vi "generate_galvo_voltages_from_fifo.vi"(0 "resonant trigger":bool, 1 "counter cluster in":T5, 2 "stim duration":u16=20, 3 "tracking settings":T1, 4 "scan specification":T4, 5 "scanning":bool, 6 "tracking":bool, 7 "x-y phase shift (*2^16/2*pi)":u16=16384, 9 "stim delay":i16=5) -> (10 "stim light window":bool, 11 "trigger diagnostics":T2, 12 "update tracking?":T3, 13 "counting photons?":bool, 14 "DAC voltages":T6 {"pockels" max=4095 step=1; "y" max=4095 step=1; "x" max=4095 step=1}, 15 "counter cluster out":T5, 17 "new circle":bool, 18 "fly-back acquisition phase?":bool, 19 "acquire?":bool)   [LabVIEW 2010]
uses:
  common_typedefs/DAC_voltage_tagResonantr.ctl
  counter_cluster_tagResonant.ctl
  scan_specification_tagResonant.ctl
  FPGA tracking/polar tracking settings.ctl
  <vilib>/rvi/DataTransferAndStorage/Container/XNode/niFpgaContainer.xnode
  <vilib>/rvi/DataTransferAndStorage/Container/Common/niFpgaContainerMethod.ctl
  <vilib>/rvi/DataTransferAndStorage/Container/Common/niFpgaTransferTypeControl.ctl
  <vilib>/rvi/Analysis/common/FxpNativeNode/niFpgaFxpNative.xnode
  <vilib>/rvi/interface/RandomDataEmulation/nirviRandomDataFPGAFIFO.vi
  <vilib>/rvi/interface/RandomDataEmulation/niFpgaRandomDataHandleErrors.vi
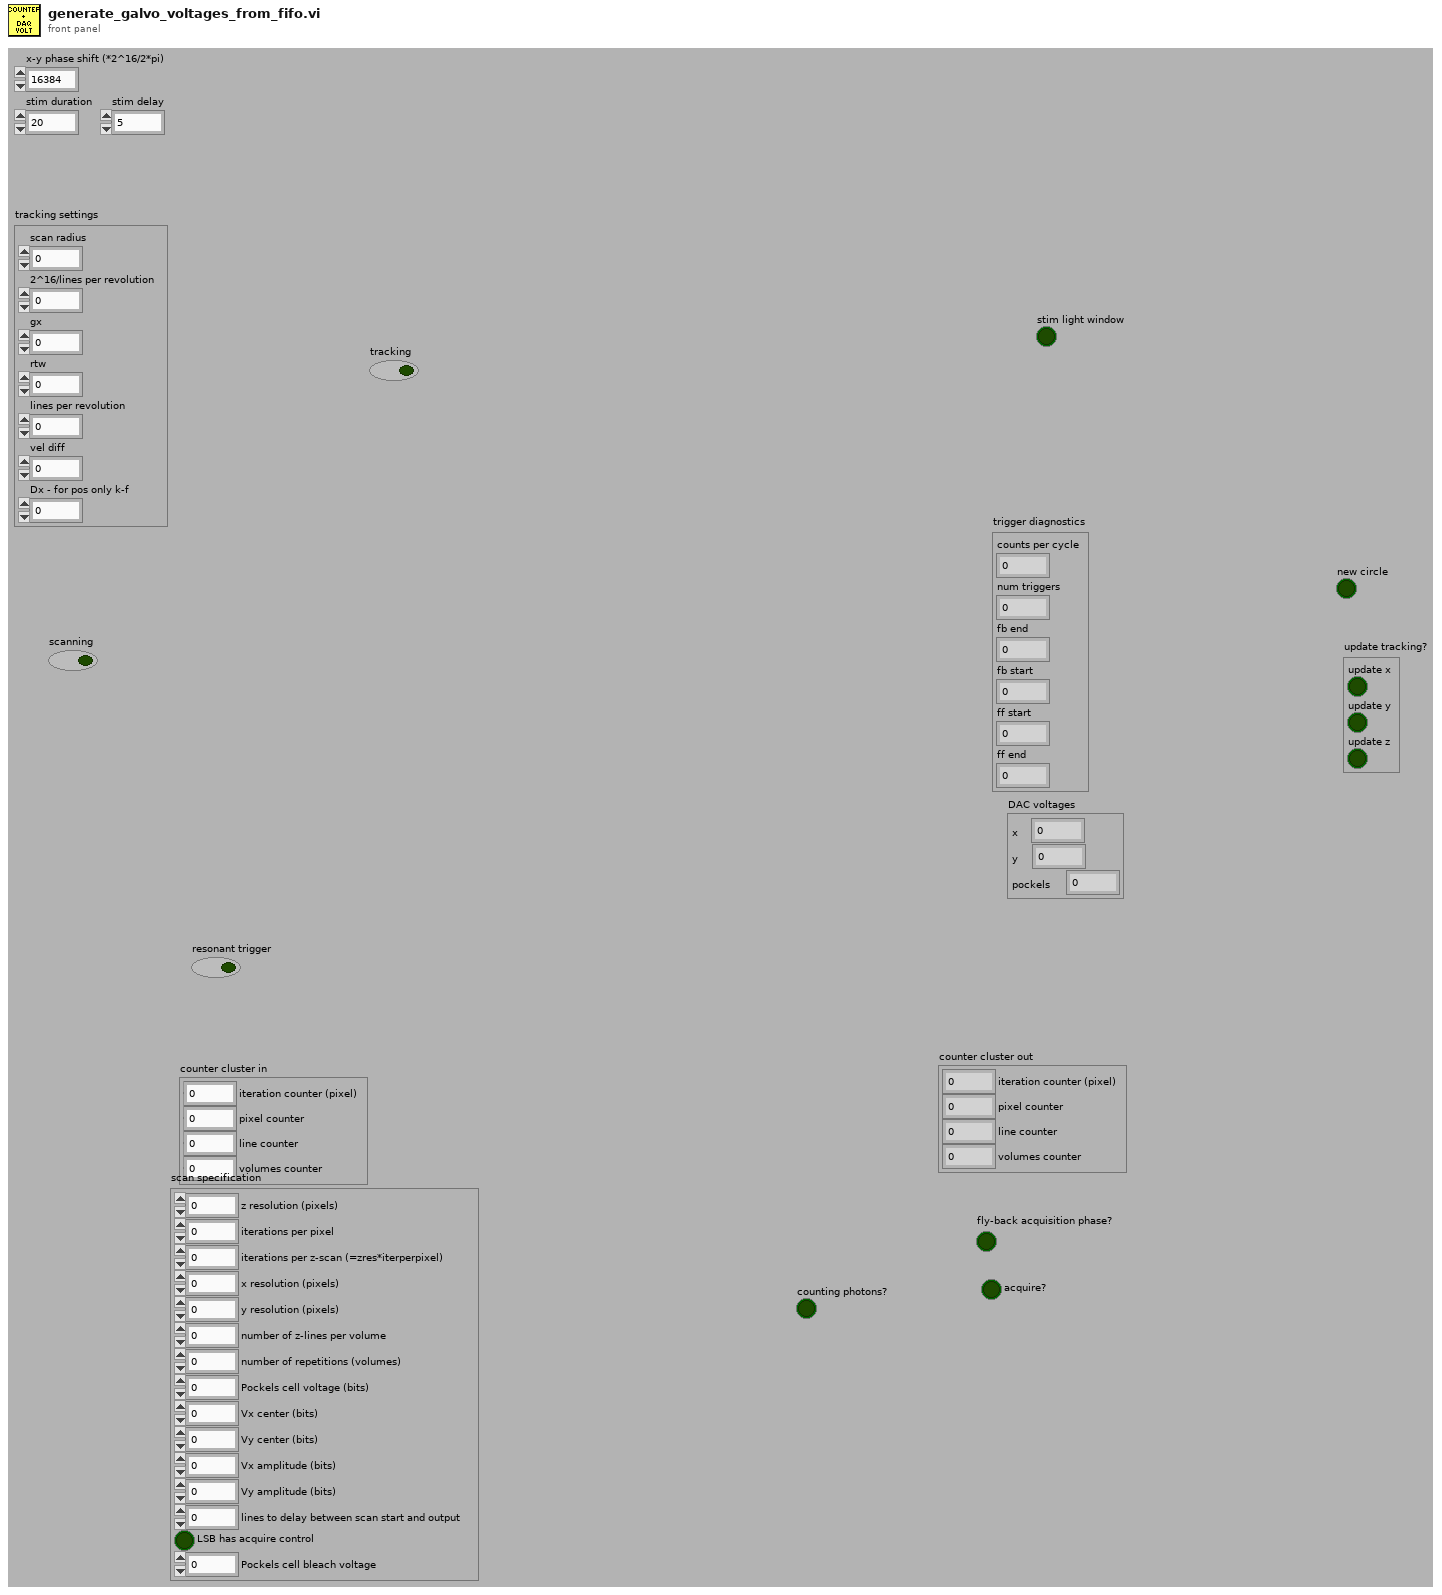
[diagram p1: front panel]
types:
  T1 = typedef "polar tracking settings.ctl" = cluster{"scan radius":u16, "2^16/lines per revolution":u16, "gx":fxp<+,16,8>, "rtw":fxp<+,16,26>, "lines per revolution":u8, "vel diff":fxp<+,24,-22>, "Dx - for pos only k-f":fxp<+,32,19>}
  T2 = cluster{"counts per cycle":u16, "num triggers":u32, "fb end":u16, "fb start":u16, "ff start":u16, "ff end":u16}
  T3 = cluster{"update x":bool, "update y":bool, "update z":bool}
  T4 = typedef "scan_specification_tagResonant.ctl" = cluster{"z resolution (pixels)":u16, "iterations per pixel":u16, "iterations per z-scan (=zres*iterperpixel)":u16, "x resolution (pixels)":u16, "y resolution (pixels)":u16, "number of z-lines per volume":u16, "number of repetitions (volumes)":i32, "Pockels cell voltage (bits)":i16, "Vx center (bits)":i16, "Vy center (bits)":i16, "Vx amplitude (bits)":i16, "Vy amplitude (bits)":i16, "lines to delay between scan start and output":u16, "LSB has acquire control":bool, "Pockels cell bleach voltage":i16}
  T5 = typedef "counter_cluster_tagResonant.ctl" = cluster{"iteration counter (pixel)":u16, "pixel counter":u16, "line counter":i16, "volumes counter":u16}
  T6 = typedef "DAC_voltage_tagResonantr.ctl" = cluster{"x":i16, "y":i16, "pockels":i16}
  T7 = typedef "niFpgaContainerMethod.ctl" = enum16{"<none>", "write", "read", "clear", "getNumberOfElementsToWrite", "getNumberOfElementsToRead", "enable", "disable", "flushAndDisable", "getStreamState", "readA", "readB", "dramWrite", "dramWriteWithByteEnables", "dramRequestData", "dramRetrieveData"}
  T8 = typedef "niFpgaTransferTypeControl.ctl" = enum16{"Target-Scoped", "Host to Target - DMA", "Target to Host - DMA", "Peer to Peer Reader", "Peer to Peer Writer", "Bidirectional"}
  T9 = cluster{"crossing":bool, "crossing":bool, "crossing":bool}
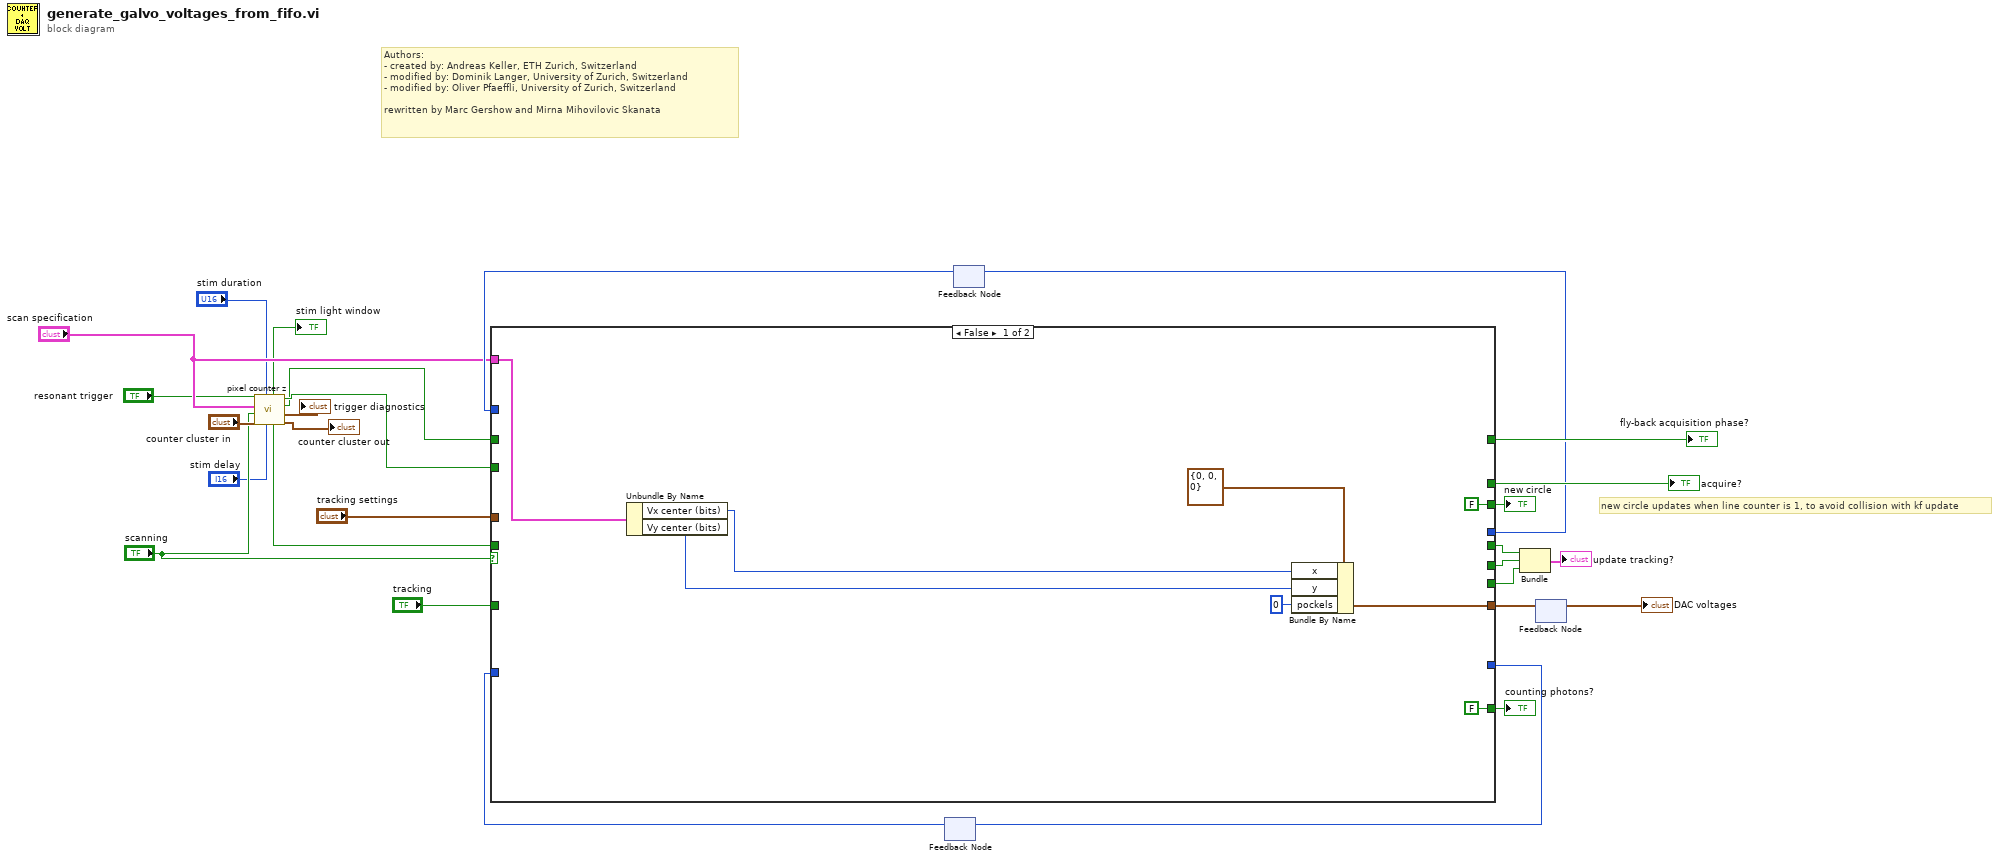
[diagram p0: block diagram]
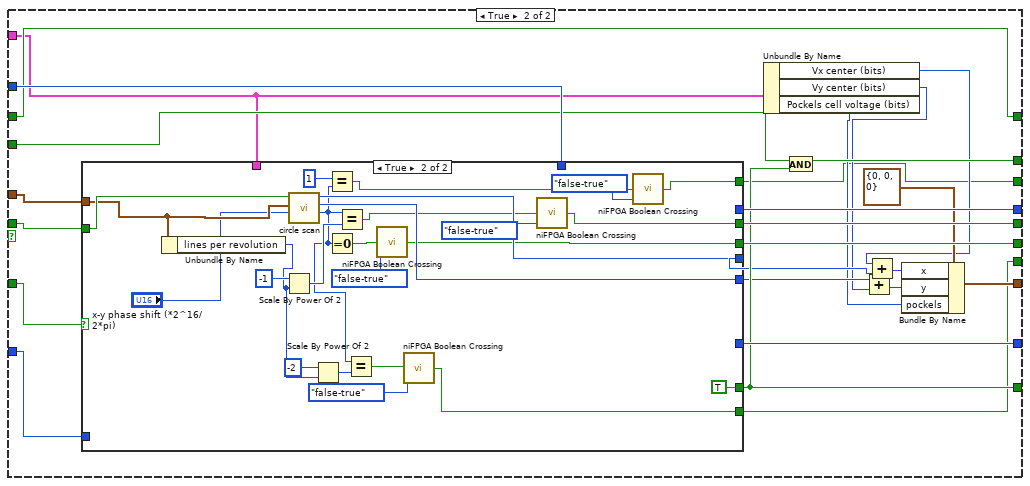
[diagram p2: hidden frame]
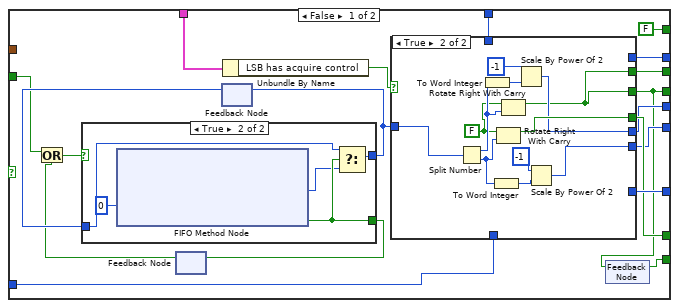
[diagram p3: hidden frame]
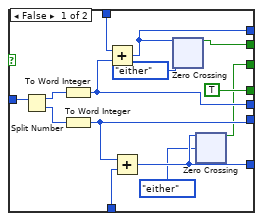
[diagram p4: hidden frame]
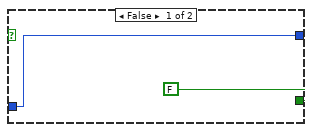
[diagram p5: hidden frame]
diagram:
  # "new circle updates when line counter is 1, to avoid collision with kf update"
  # "Authors: \n- created by: Andreas Keller, ETH Zurich, Switzerland\n- modified by: Dominik Langer, University of Zurich, Switzerland\n- modified by: Oliver Pfaeffli, University of Zurich, Switzerland\n\nrewritten by Marc Gershow and Mirna Mihovilovic Skanata"
  n1 = call "pixel counter z.vi"("stim delay"="stim delay", "stim duration"="stim duration", "counter cluster in"="counter cluster in", "scanning"="scanning", "scan specification"="scan specification", "tag lens trigger"="resonant trigger") -> ("counter cluster out"=→"counter cluster out":T5, "trigger diagnostics"=→"trigger diagnostics":T2, "fly back"=w10:bool, "acquire"=w11:bool, "new line"=w12:bool, "stim light window"=→"stim light window":bool)
  n2 = feedback #1() -> (w24:i16)  [unwired: 1 in]
  n3 = feedback #2() -> (w22:i16)  [unwired: 1 in]
  n4 = case shown="False" "scanning" {
    tunnel: [w31 w61] -> w28
    tunnel: [_ w51] -> w27
    tunnel: [_ w54] -> w26
    tunnel: [_ w60] -> w23
    tunnel: [_ w59] -> w25
    tunnel: w24 -> [_ w57]
    tunnel: w22 -> [_ w58]
    tunnel: [_ w56] -> w19
    tunnel: [_ w55] -> w20
    tunnel: [FALSE ("lsb carry out") w53] -> w21
    tunnel: "scan specification" -> [w34 w50]
    tunnel: w12 -> [_ w49]
    tunnel: w11 -> [_ w52]
    tunnel: w10 -> [_ w51]
    tunnel: [_ w38] -> w8
    tunnel: "tracking" -> [_ w40]
    tunnel: "tracking settings" -> [_ w39]
    tunnel: [FALSE w37] -> w2
    frame False {
      n5 = Unbundle By Name(w34) -> ("Vx center (bits)"=w33:i16, "Vy center (bits)"=w32:i16)
      n6 = Bundle By Name(cluster=T6 {"x"=0, "y"=0, "pockels"=0} ("DAC voltage"), "x"=w33, "y"=w32, "pockels"=i16 0) -> (w31:T6)
    }
    frame True {
      n7 = case shown="True" w40 {
        tunnel: [w80 _] -> w60
        tunnel: [w79 _] -> w59
        tunnel: w58 -> [w78 _]
        tunnel: w57 -> [w77 _]
        tunnel: [w76 w187] -> w56
        tunnel: [w64 w190] -> w55
        tunnel: [w75 TRUE ("lsb carry out")] -> w53
        tunnel: w50 -> [w74 _]
        tunnel: w49 -> [w65 w196]
        tunnel: [w67 w199] -> w47
        tunnel: [w66 w198] -> w46
        tunnel: w39 -> [_ w195]
        tunnel: [w63 w181] -> w38
        tunnel: [FALSE w176] -> w37
        frame False {
          n8 = feedback #3() -> (w70:bool)  [unwired: 1 in]
          n9 = Or(x=w65, y=w70) -> (x .or. y?=w72:bool)
          n10 = feedback #4() -> (w73:u32)  [unwired: 1 in]
          n11 = case shown="True" w72 {
            tunnel: [w140 w144] -> w68
            tunnel: w73 -> [w140 w141]
            tunnel: [FALSE ("Timed Out?") w143] -> w71
            frame False {
            }
            frame True {
              n12 = xnode ("FIFO Method Node")("Timeout"=0) -> ("Element"=w142:u32, "Timed Out?"=w143:bool)  [unwired: 1 in, 1 out]
              n13 = Select(t=w141, s=w143, f=w142) -> (s? t:f=w144:u32)
            }
          }
          n14 = feedback-in #3(w71) -> ()
          n15 = feedback-in #4(w68) -> ()
          n16 = Unbundle By Name(w74) -> ("LSB has acquire control"=w69:bool)
          n17 = case shown="True" w69 {
            tunnel: w68 -> [w93 w138]
            tunnel: [w90 w131] -> w67
            tunnel: [w89 w135] -> w66
            tunnel: [TRUE ("lsb carry out") w133] -> w75
            tunnel: [w81 w127] -> w64
            tunnel: [w84 w127] -> w76
            tunnel: [w86 _] -> w80
            tunnel: [w83 _] -> w79
            tunnel: w78 -> [w88 _]
            tunnel: w77 -> [w87 _]
            frame False {
              n18 = Split Number(x=w93) -> (hi(x)=w92:u16, lo(x)=w91:u16)
              n19 = To Word Integer(number=w92) -> (16bit integer=w90:i16)
              n20 = To Word Integer(number=w91) -> (16bit integer=w89:i16)
              n21 = Add(x=w88, y=w90) -> (x+y=w86:i16)
              n22 = Add(x=w89, y=w87) -> (x+y=w83:i16)
              n23 = xnode ("Zero Crossing")("direction"=enum8{"either", "minus-plus", "plus-minus"}."either", "input"=w86) -> ("crossing"=w84:bool)  [unwired: 1 in]
              n24 = xnode ("Zero Crossing")("direction"=enum8{"either", "minus-plus", "plus-minus"}."either", "input"=w83) -> ("crossing"=w81:bool)  [unwired: 1 in]
            }
            frame True {
              w128 = FALSE ("carry")
              n25 = Split Number(x=w138) -> (hi(x)=w129:u16, lo(x)=w137:u16)
              n26 = To Word Integer(number=w129) -> (16bit integer=w132:i16)
              n27 = To Word Integer(number=w137) -> (16bit integer=w134:i16)
              n28 = Rotate Right With Carry(2:w137, 3:w128) -> (1:w133:bool)  [unwired: 1 out]
              n29 = Rotate Right With Carry(2:w129, 3:w128) -> (1:w127:bool)  [unwired: 1 out]
              n30 = Scale By Power Of 2(n=-1, x=w132) -> (x*2^n=w131:i16)
              n31 = Scale By Power Of 2(n=-1, x=w134) -> (x*2^n=w135:i16)
            }
          }
          n32 = feedback-in #5(w64) -> ()
          n33 = feedback #5() -> (w63:bool)  [unwired: 1 in]
        }
        frame True {
          n34 = Unbundle By Name(w195) -> ("lines per revolution"=w185:u8)
          n35 = Scale By Power Of 2(n=-1, x=w185) -> (x*2^n=w193:u8)
          n36 = call "circle scan.vi"("x-y phase shift (*2^16/2*pi)"="x-y phase shift (*2^16/2*pi)", "tracking settings"=w195, "new line"=w196) -> ("line counter"=w179:u8, "y value"=w198:i16, "x value"=w199:i16)  [unwired: 6 in]
          n37 = Scale By Power Of 2(n=-2, x=w185) -> (x*2^n=w184:u8)
          n38 = Equal?(x=u8 1, y=w179) -> (x = y?=w177:bool)
          n39 = Equal To 0?(x=w179) -> (x = 0?=w192:bool)
          n40 = Equal?(x=w179, y=w193) -> (x = y?=w188:bool)
          n41 = Equal?(x=w179, y=w184) -> (x = y?=w182:bool)
          n42 = call <vilib>:"niFPGA Boolean Crossing.vi"("input"=w192, "direction"=enum8{"either", "false-true", "true-false"}."false-true") -> ("crossing"=w190:bool)  [unwired: 7 in]
          n43 = call <vilib>:"niFPGA Boolean Crossing.vi"("input"=w182, "direction"=enum8{"either", "false-true", "true-false"}."false-true") -> ("crossing"=w181:bool)  [unwired: 7 in]
          n44 = call <vilib>:"niFPGA Boolean Crossing.vi"("input"=w188, "direction"=enum8{"either", "false-true", "true-false"}."false-true") -> ("crossing"=w187:bool)  [unwired: 7 in]
          n45 = call <vilib>:"niFPGA Boolean Crossing.vi"("input"=w177, "direction"=enum8{"either", "false-true", "true-false"}."false-true") -> ("crossing"=w176:bool)  [unwired: 7 in]
        }
      }
      n46 = Unbundle By Name(w50) -> ("Vx center (bits)"=w44:i16, "Vy center (bits)"=w42:i16, "Pockels cell voltage (bits)"=w41:i16)
      n47 = And(x=w52, y=w53) -> (x .and. y?=w54:bool)
      n48 = Add(x=w46, y=w42) -> (x+y=w43:i16)
      n49 = Add(x=w44, y=w47) -> (x+y=w45:i16)
      n50 = Bundle By Name(cluster=T6 {"x"=0, "y"=0, "pockels"=0} ("DAC voltage"), "x"=w45, "y"=w43, "pockels"=w41) -> (w61:T6)
    }
  }
  "acquire?" <- w26
  "fly-back acquisition phase?" <- w27
  "counting photons?" <- w21
  "new circle" <- w2
  n51 = feedback-in #1(w25) -> ()
  n52 = feedback-in #2(w23) -> ()
  n53 = Bundle("crossing"=w19, "crossing"=w20, "crossing"=w8) -> (→"update tracking?":T9)  [unwired: 1 in]
  n54 = feedback-in #6(w28) -> ()
  n55 = feedback #6() -> (→"DAC voltages":T6)  [unwired: 1 in]
